vi "Sub-Panel Drop-In.vi"(11 "SubPanel in":refnum<vi>) -> ()   [LabVIEW 2020]
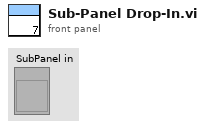
[diagram p1: front panel]
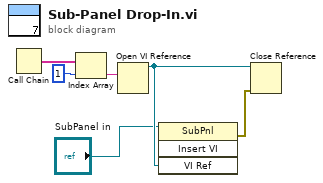
[diagram p0: block diagram]
diagram:
  n1 = Call Chain() -> (call chain=w4:string[])
  n2 = Index Array(array=w4, index=1) -> (element=w6:string)
  n3 = Open VI Reference(vi path=w6) -> (vi reference=w2:refnum<vi>)  [unwired: 5 in, 1 out]
  n4 = invoke class="SubPnl" method="Insert VI"(reference="SubPanel in", "VI Ref"=w2) -> (error out=w3:errorcluster)  [unwired: 2 in, 3 out]
  n5 = Close Reference(reference=w2, error in (no error)=w3) -> ()  [unwired: 1 out]
